vi "bin_level_Lalit.vi"() -> ()   [LabVIEW 2014]
uses:
  <vilib>/Instr/_visa.llb/VISA Configure Serial Port (Instr).vi
panel:
  out "BIN4":dbl(slide) scale=0.0..100.0
  out "BIN3":dbl(slide) scale=0.0..100.0
  out "BIN2":dbl(slide) scale=0.0..100.0
  out "BIN1":dbl(slide) scale=0.0..100.0
  in  "stop bits (10: 1 bit)":u16(ring)=10 items=["1.0"=10, "1.5"=15, "2.0"=20]
  in  "parity (0:none)":enum16{"None", "Odd", "Even", "Mark", "Space"}(ring)
  in  "data bits (8)":u16=8 min=5 max=8 step=1
  in  "baud rate (9600)":u32=9600
  out "BIN4(mV)":dbl
  out "BIN3(mV)":dbl
  out "BIN2(mV)":dbl
  out "BIN1(mV)":dbl
  out "BIN4":string
  out "BIN3":string
  out "BIN2":string
  in  "STOP":bool
  out "BIN1":string
  out "read buffer":string
  in  "Byte count":u32
  in  "VISA resource name":refnum<visa-resource-name>
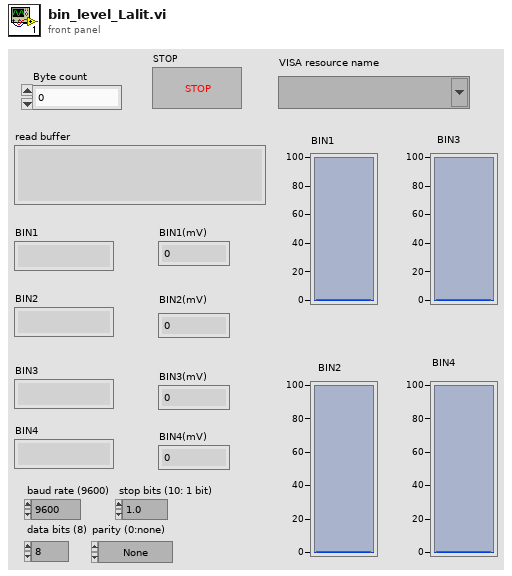
[diagram p1: front panel]
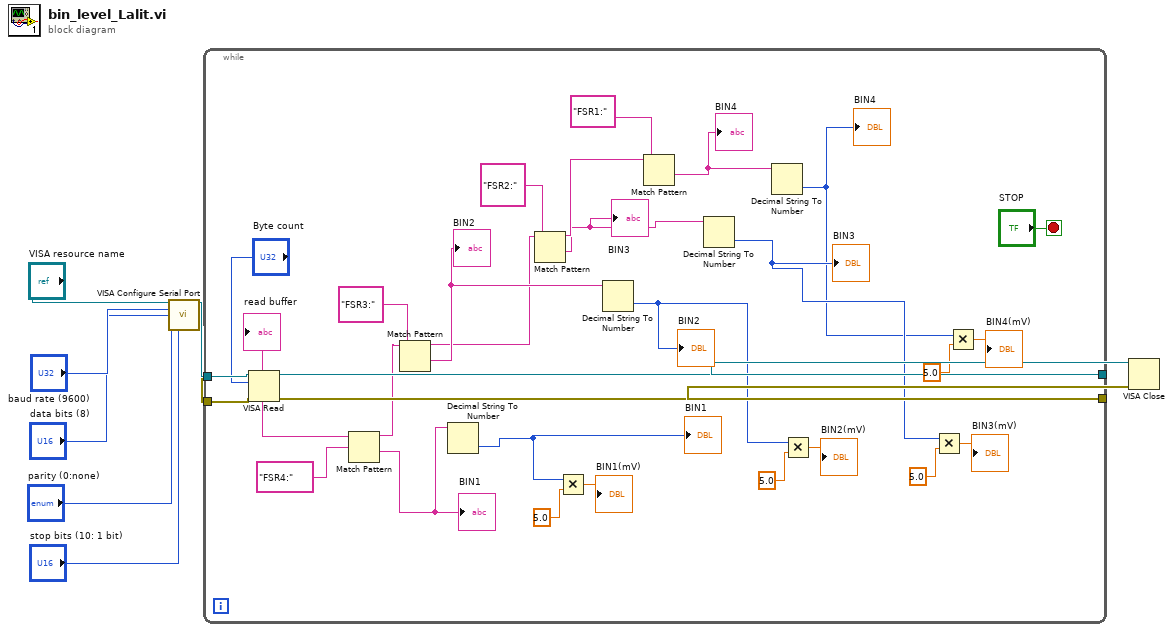
[diagram p0: block diagram]
diagram:
  n1 = call-poly "VISA Configure Serial Port"("VISA resource name"="VISA resource name", "baud rate (9600)"="baud rate (9600)", "data bits (8)"="data bits (8)", "parity (0:none)"="parity (0:none)", "stop bits (10: 1 bit)"="stop bits (10: 1 bit)") -> ("VISA resource name out"=w8:refnum<visa-resource-name>, "error out"=w7:errorcluster)  [unwired: 9 in]
  n2 = while {
    tunnel: w8 -> [w39]
    tunnel: w7 -> [w38]
    tunnel: [w33] -> w6
    tunnel: [w32] -> w5
    stop <- "STOP" stop-if-true
    n3 = VISA Read(VISA resource name=w39, byte count="Byte count", error in (no error)=w38) -> (VISA resource name out=w32:refnum<visa-resource-name>, read buffer=w36:string, error out=w33:errorcluster)  [unwired: 1 out]
    "read buffer" <- w36
    n4 = Match Pattern(string=w36, regular expression="FSR4:") -> (before substring=w31:string, after substring=w34:string)  [unwired: 1 in, 2 out]
    "BIN1" <- w34
    n5 = Match Pattern(string=w31, regular expression="FSR3:") -> (before substring=w23:string, after substring=w26:string)  [unwired: 1 in, 2 out]
    "BIN2" <- w26
    n6 = Decimal String To Number(string=w34) -> (number=w14:i32)  [unwired: 2 in, 1 out]
    "BIN1" <- w14
    n7 = Match Pattern(string=w23, regular expression="FSR2:") -> (before substring=w30:string, after substring=w25:string)  [unwired: 1 in, 2 out]
    "BIN3" <- w25
    n8 = Multiply(x=w14, y=5.0) -> (x*y=→"BIN1(mV)":dbl)
    n9 = Decimal String To Number(string=w26) -> (number=w13:i32)  [unwired: 2 in, 1 out]
    "BIN2" <- w13
    n10 = Match Pattern(string=w30, regular expression="FSR1:") -> (after substring=w24:string)  [unwired: 1 in, 3 out]
    "BIN4" <- w24
    n11 = Decimal String To Number(string=w25) -> (number=w12:i32)  [unwired: 2 in, 1 out]
    "BIN3" <- w12
    n12 = Decimal String To Number(string=w24) -> (number=w11:i32)  [unwired: 2 in, 1 out]
    "BIN4" <- w11
    n13 = Multiply(x=w13, y=5.0) -> (x*y=→"BIN2(mV)":dbl)
    n14 = Multiply(x=w12, y=5.0) -> (x*y=→"BIN3(mV)":dbl)
    n15 = Multiply(x=w11, y=5.0) -> (x*y=→"BIN4(mV)":dbl)
  }
  n16 = VISA Close(VISA resource name=w5, error in (no error)=w6) -> ()  [unwired: 1 out]
